vi "New-LUTindx.vi"(6 "centroid":dbl[](array[numeric]), 7 "exit angles":dbl[](array[numeric]), 9 "center":dbl[](array[numeric]), 10 "rad":dbl, 11 "LUT":dbl[][](array[numeric])) -> (3 "output":dbl[](array[numeric]) format="%.2f")   [LabVIEW 2019]
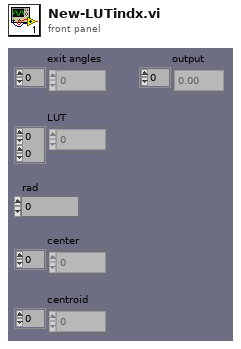
[diagram p1: front panel]
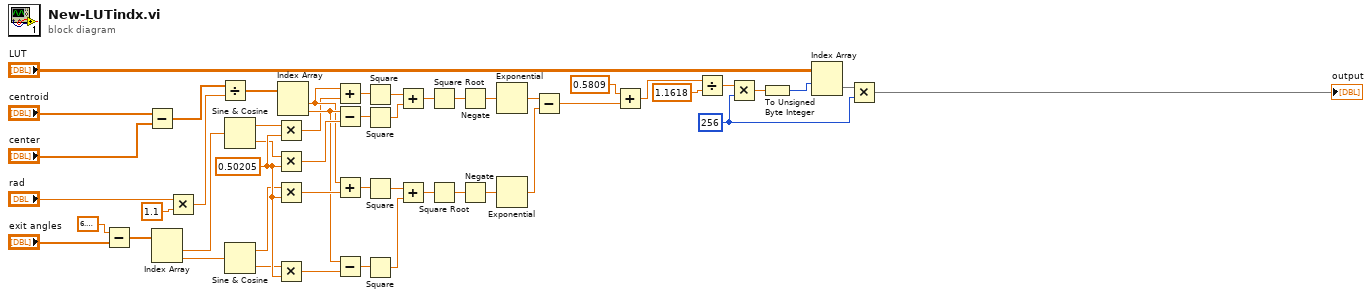
[diagram p0: block diagram]
diagram:
  w29 = 0.50205
  w49 = 256
  n1 = Subtract(x=6.283185307179586, y="exit angles") -> (x-y=w46:dbl[])
  n2 = Subtract(x="centroid", y="center") -> (x-y=w8:dbl[])
  n3 = Index Array(array=w46) -> (element #1=w43:dbl, element #2=w44:dbl)  [unwired: 2 in]
  n4 = Multiply(x="rad", y=1.1) -> (x*y=w37:dbl)
  n5 = Divide(x=w8, y=w37) -> (x/y=w9:dbl[])
  n6 = Sine & Cosine(0:w43) -> (1:w4:dbl, 2:w5:dbl)
  n7 = Sine & Cosine(0:w44) -> (1:w6:dbl, 2:w7:dbl)
  n8 = Multiply(x=w4, y=w29) -> (x*y=w10:dbl)
  n9 = Multiply(x=w5, y=w29) -> (x*y=w42:dbl)
  n10 = Multiply(x=w6, y=w29) -> (x*y=w27:dbl)
  n11 = Multiply(x=w7, y=w29) -> (x*y=w28:dbl)
  n12 = Index Array(array=w9) -> (element #1=w25:dbl, element #2=w26:dbl)  [unwired: 2 in]
  n13 = Add(x=w25, y=w10) -> (x+y=w11:dbl)
  n14 = Subtract(x=w26, y=w42) -> (x-y=w13:dbl)
  n15 = Add(x=w25, y=w27) -> (x+y=w23:dbl)
  n16 = Subtract(x=w26, y=w28) -> (x-y=w24:dbl)
  n17 = Square(x=w11) -> (x^2=w14:dbl)
  n18 = Square(x=w13) -> (x^2=w12:dbl)
  n19 = Square(x=w23) -> (x^2=w19:dbl)
  n20 = Square(x=w24) -> (x^2=w18:dbl)
  n21 = Add(x=w14, y=w12) -> (x+y=w15:dbl)
  n22 = Add(x=w19, y=w18) -> (x+y=w20:dbl)
  n23 = Square Root(x=w15) -> (sqrt(x)=w16:dbl)
  n24 = Square Root(x=w20) -> (sqrt(x)=w21:dbl)
  n25 = Negate(x=w16) -> (-x=w17:dbl)
  n26 = Negate(x=w21) -> (-x=w22:dbl)
  n27 = Exponential(1:w17) -> (0:w39:dbl)
  n28 = Exponential(1:w22) -> (0:w40:dbl)
  n29 = Subtract(x=w39, y=w40) -> (x-y=w33:dbl)
  n30 = Add(x=0.5809, y=w33) -> (x+y=w35:dbl)
  n31 = Divide(x=w35, y=1.1618) -> (x/y=w41:dbl)
  n32 = Multiply(x=w41, y=w49) -> (x*y=w2:dbl)
  n33 = To Unsigned Byte Integer(number=w2) -> (unsigned 8bit integer=w3:u8)
  n34 = Index Array(array="LUT", index (row)=w3) -> (element=w48:dbl[])  [unwired: 1 in]
  n35 = Multiply(x=w48, y=w49) -> (x*y=→"output":dbl[])
